vi "Authorize.vi"(6 "timeout (ms) [0: default]":i32, 8 "error in (no error)":errorcluster, 10 "State Parameter":string, 11 "Oauth2 in":refnum<class "Oauth2.lvclass">) -> (0 "error out":errorcluster, 2 "Access Token":string, 3 "Oauth2 out":refnum<class "Oauth2.lvclass">)   [LabVIEW 2013, in "Oauth2.lvclass"]
uses:
  Oauth2.lvclass
  OAuthToken/OAuth2 Token Element -- enum.ctl
  Oauth2.lvclass/Oauth2.ctl
  <vilib>/LabVIEW Open Source Project/OpenURI/uri/URI.lvclass/URI.ctl
  <vilib>/LabVIEW Open Source Project/OpenURI/uri/URI.lvclass
  OAuthToken/OAuthAccessToken.lvclass
  <vilib>/LabVIEW Open Source Project/Connection/Connection.TCP/Connection.TCP.lvclass
  <vilib>/LabVIEW Open Source Project/Connection/Connection/Connection.lvclass
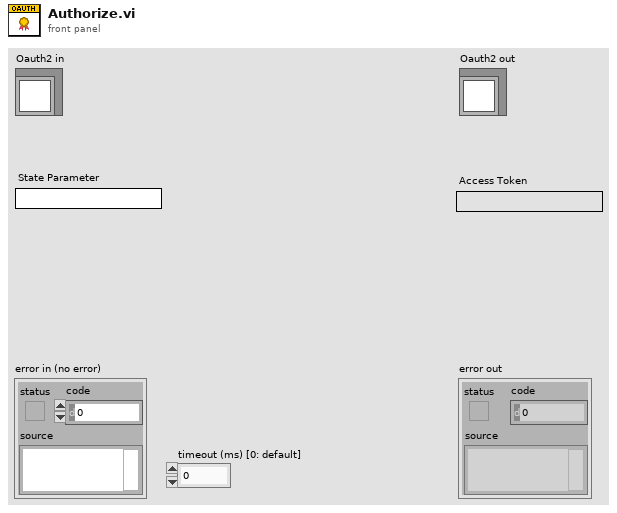
[diagram p1: front panel]
types:
  T1 = typedef "OAuthAccessToken.lvclass/OAuth2 Token Element -- enum.ctl" = enum16{"client_id", "client_secret", "response_type", "scope", "redirect_uri", "error", "error_description", "error_uri", "grant_type", "code", "access_token", "token_type", "expires_in", "username", "password", "refresh_token", "code_challenge", "code_challenge_method", "endpoint element"}
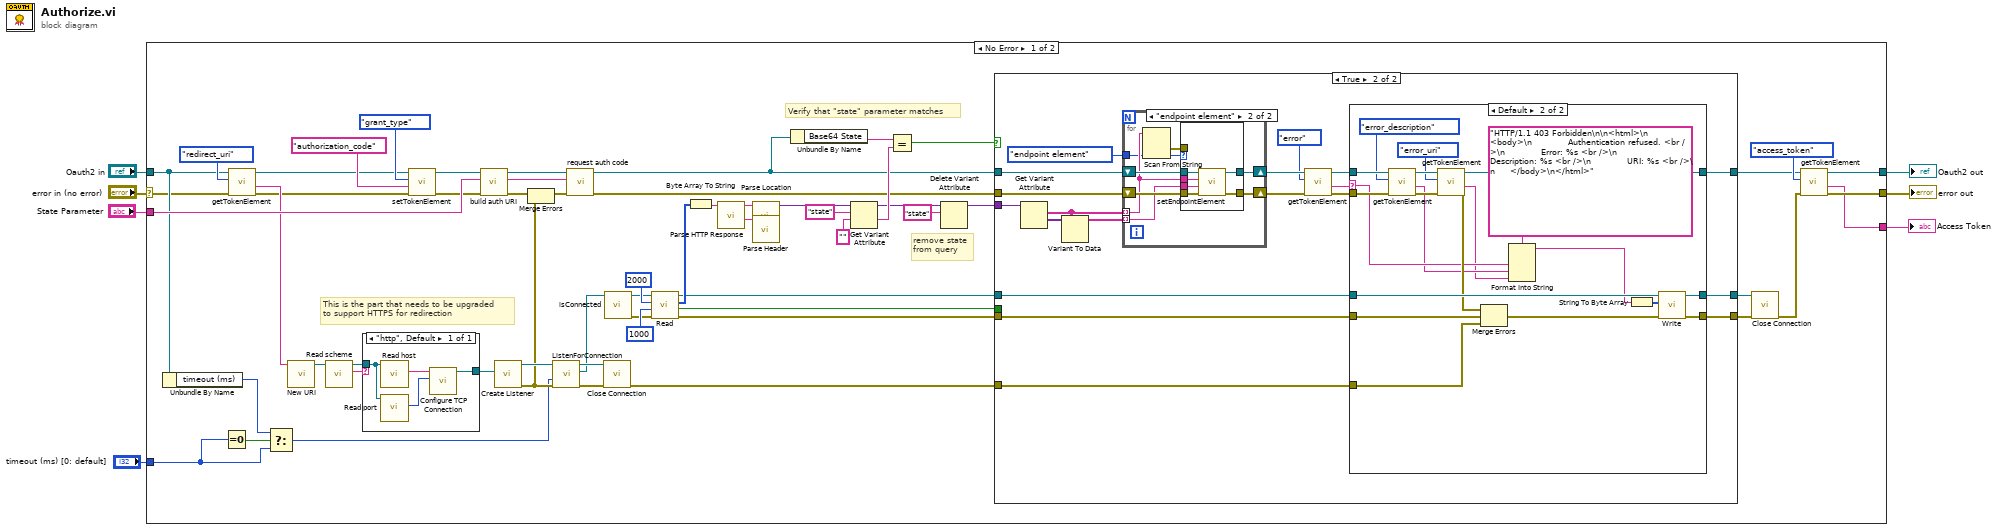
[diagram p0: block diagram]
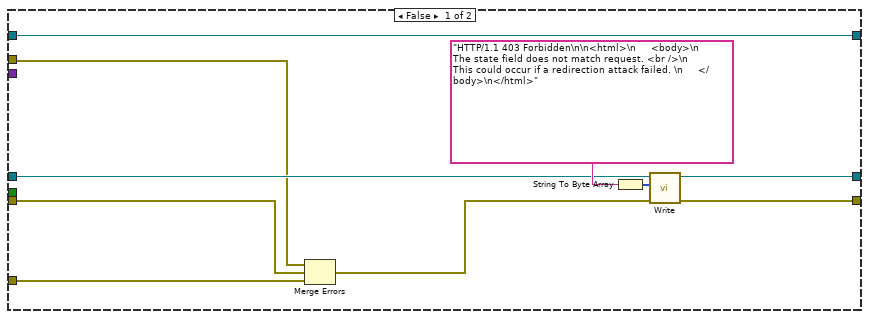
[diagram p2: hidden frame]
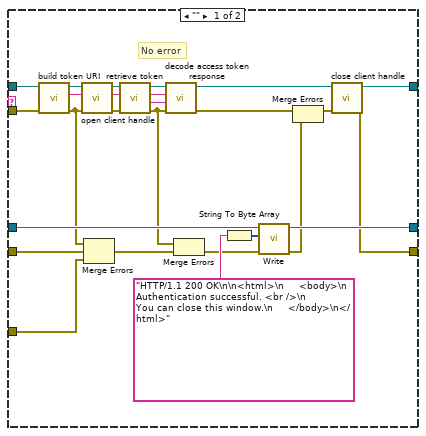
[diagram p3: hidden frame]
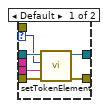
[diagram p4: hidden frame]
diagram:
  n1 = case shown="No Error" "error in (no error)" {
    selector: "error in (no error)" -> [w31 w168]
    tunnel: [w35 w168] -> w6
    tunnel: [w37 w167] -> w4
    tunnel: "Oauth2 in" -> [w32 w167]
    tunnel: "State Parameter" -> [w64 _]
    tunnel: [w27 _] -> w2
    tunnel: "timeout (ms) [0: default]" -> [w10 _]
    frame No Error {
      # "This is the part that needs to be upgraded\nto support HTTPS for redirection"
      # "remove state\nfrom query"
      # "Verify that \"state\" parameter matches"
      n2 = Unbundle By Name(w32) -> ("timeout (ms)"=w43:i32)
      n3 = Equal To 0?(x=w10) -> (x = 0?=w44:bool)
      n4 = call "getTokenElement.vi"("error in (no error)"=w31, "Token element"=OAuth2_Token_Element_--_enum."redirect_uri", "Oauth2 in"=w32) -> ("error out"=w8:errorcluster, "Value"=w30:string, "Oauth2 out"=w9:refnum<class "Oauth2.lvclass">)  [unwired: 5 in, 1 out]
      n5 = Select(t=w43, s=w44, f=w10) -> (s? t:f=w42:i32)
      n6 = call <vilib>:"New URI.vi"("URI"=w30) -> ("URI"=w29:refnum<class "URI.lvclass">)  [unwired: 9 in, 1 out]
      n7 = call <vilib>:"Read scheme.vi"("URI in"=w29) -> ("scheme"=w66:string, "URI out"=w65:refnum<class "URI.lvclass">)  [unwired: 8 in, 1 out]
      n8 = case shown="\"http\", Default" w66 {
        tunnel: w65 -> [w163]
        tunnel: [w164] -> w55
        frame "http", Default {
          n9 = call <vilib>:"Read host.vi"("URI in"=w163) -> ("host"=w166:string)  [unwired: 8 in, 2 out]
          n10 = call <vilib>:"Read port.vi"("URI in"=w163) -> ("port"=w165:u16)  [unwired: 8 in, 2 out]
          n11 = call <vilib>:"Configure TCP Connection.vi"("remote port (80)"=w165, "address (localhost)"=w166) -> ("Connection.TCP"=w164:refnum<class "Connection.TCP.lvclass">)  [unwired: 8 in, 1 out]
        }
      }
      n12 = call "setTokenElement.vi"("error in (no error)"=w8, "Value"="authorization_code", "Token element"=OAuth2_Token_Element_--_enum."grant_type", "Oauth2 in"=w9) -> ("error out"=w11:errorcluster, "Oauth2 out"=w12:refnum<class "Oauth2.lvclass">)  [unwired: 6 in]
      n13 = call "build auth URI.vi"("error in (no error)"=w11, "State Parameter"=w64, "Oauth2 in"=w12) -> ("error out"=w49:errorcluster, "Authorization Request URI"=w51:string, "Oauth2"=w50:refnum<class "Oauth2.lvclass">)  [unwired: 6 in]
      n14 = call <vilib>:"Create Listener.vi"("Connection Configuration"=w55) -> ("error out"=w53:errorcluster, "Listener"=w61:refnum<class "Connection.lvclass">)  [unwired: 9 in]
      n15 = Merge Errors(w49, w53) -> (w52:errorcluster)
      n16 = call <vilib>:"ListenForConnection.vi"("error in (no error)"=w53, "timeout (2000 ms)"=w42, "Listener"=w61) -> ("error out"=w63:errorcluster, "Connection"=w58:refnum<class "Connection.lvclass">, "Listener out"=w60:refnum<class "Connection.lvclass">)  [unwired: 5 in, 1 out]
      n17 = call-dynamic "request auth code.vi"("error in (no error)"=w52, "Request URI"=w51, "Oauth2 in"=w50) -> ("error out"=w18:errorcluster, "Oauth2 out"=w19:refnum<class "Oauth2.lvclass">)  [unwired: 7 in]
      n18 = call <vilib>:"Close Connection.vi"("error in (no error)"=w63, "Connection in"=w60) -> ("error out"=w46:errorcluster)  [unwired: 8 in, 1 out]
      n19 = call <vilib>:"isConnected.vi"("Connection in"=w58) -> ("error out"=w56:errorcluster, "Connection out"=w57:refnum<class "Connection.lvclass">)  [unwired: 8 in, 1 out]
      n20 = call <vilib>:"Read.vi"("error in (no error)"=w56, "timeout (2000 ms)"=1000 ("bytes to read (100)"), "bytes to read (100)"=2000, "TCPConnection in"=w57) -> ("error out"=w45:errorcluster, "timed out"=w38:bool, "Bytes"=w54:u8[], "TCPConnection out"=w47:refnum<class "Connection.lvclass">)  [unwired: 3 in, 1 out]
      n21 = Byte Array To String(unsigned byte array=w54) -> (string=w26:string)
      n22 = call "Parse HTTP Response.vi"("HTTP Response"=w26) -> ("Header"=w25:string, "Location"=w24:string)  [unwired: 5 in, 4 out]
      n23 = call "Parse Location.vi"("Location"=w24) -> ("Query Parameters"=w23:variant)  [unwired: 10 in]
      n24 = call "Parse Header.vi"("HTTP Header"=w25) -> ()  [unwired: 10 in, 1 out]
      n25 = Unbundle By Name(w19) -> ("Base64 State"=w40:string)
      n26 = Get Variant Attribute(Variant=w23, name="state", default value (empty Variant)="") -> (duplicate Variant=w17:variant, value=w20:string)  [unwired: 1 in, 2 out]
      n27 = Equal?(x=w40, y=w20) -> (x = y?=w39:bool)
      n28 = Delete Variant Attribute(6:"state", 7:w17) -> (3:w16:variant)  [unwired: 1 in, 2 out]
      n29 = case shown="True" w39 {
        tunnel: w19 -> [w68 w89]
        tunnel: w18 -> [w67 w88]
        tunnel: [w73 w95] -> w48
        tunnel: w47 -> [w74 w94]
        tunnel: w46 -> [w71 w93]
        tunnel: w45 -> [w70 w92]
        tunnel: [w68 w91] -> w28
        tunnel: [w72 w90] -> w41
        tunnel: w38 -> [_ _]
        tunnel: w16 -> [_ w83]
        frame False {
          n30 = Merge Errors(w67, w70, w71) -> (w69:errorcluster)
          n31 = String To Byte Array(string="HTTP/1.1 403 Forbidden\n\n<html>\n     <body>\n           The state field does not match request. <br />\n           This could occur if a redirection attack failed. \n     </body>\n</html>" ("regular expression")) -> (unsigned byte array=w76:u8[])
          n32 = call <vilib>:"Write.vi"("error in (no error)"=w69, "Bytes"=w76, "Connection in"=w74) -> ("error out"=w72:errorcluster, "Connection"=w73:refnum<class "Connection.lvclass">)  [unwired: 7 in]
        }
        frame True {
          n33 = Get Variant Attribute(Variant=w83) -> (names=w84:string[], values=w86:variant[])  [unwired: 3 in, 2 out]
          n34 = Variant To Data(type=w84, Variant=w86) -> (data=w85:string[])  [unwired: 1 in, 1 out]
          n35 = for {
            shift-right: [w148] -> w82
            shift-left: w89 -> [w149]
            shift-right: [w145] -> w80
            shift-left: w88 -> [w147]
            tunnel: w84 -> [w143] mode=indexing
            tunnel: w85 -> [w146] mode=indexing
            tunnel: OAuth2_Token_Element_--_enum."endpoint element" ("Token element") -> [w142]
            n36 = Scan From String(input string=w143, default 1=w142) -> (error out=w144:errorcluster, output 1=w150:T1)  [unwired: 3 in, 2 out]
            n37 = case shown="\"endpoint element\"" w150 {
              selector: w150 -> [w154 _]
              tunnel: w149 -> [w156 w162]
              tunnel: [w155 w161] -> w148
              tunnel: w147 -> [w153 w160]
              tunnel: w146 -> [w152 w158]
              tunnel: [w151 w159] -> w145
              tunnel: w144 -> [_ _]
              tunnel: w143 -> [_ w157]
              frame Default {
                n38 = call "setTokenElement.vi"("error in (no error)"=w153, "Value"=w152, "Token element"=w154, "Oauth2 in"=w156) -> ("error out"=w151:errorcluster, "Oauth2 out"=w155:refnum<class "Oauth2.lvclass">)  [unwired: 6 in]
              }
              frame "endpoint element" {
                n39 = call "setEndpointElement.vi"("error in (no error)"=w160, "Value"=w158, "Endpoint Name"=w157, "Oauth2 in"=w162) -> ("error out"=w159:errorcluster, "Oauth2 out"=w161:refnum<class "Oauth2.lvclass">)  [unwired: 6 in]
              }
            }
          }
          n40 = call "getTokenElement.vi"("error in (no error)"=w80, "Token element"=OAuth2_Token_Element_--_enum."error", "Oauth2 in"=w82) -> ("error out"=w79:errorcluster, "Value"=w77:string, "Oauth2 out"=w81:refnum<class "Oauth2.lvclass">)  [unwired: 5 in, 1 out]
          n41 = case shown="Default" w77 {
            selector: w77 -> [_ w126]
            tunnel: [w121 w141] -> w95
            tunnel: w94 -> [w118 w139]
            tunnel: w93 -> [w117 w138]
            tunnel: w92 -> [w116 w137]
            tunnel: [w109 w131] -> w91
            tunnel: [w98 w136] -> w90
            tunnel: w81 -> [w97 w134]
            tunnel: w79 -> [w96 w129]
            frame "" {
              # "No error"
              n42 = call-dynamic "build token URI.vi"("error in (no error)"=w96, "Oauth2 in"=w97) -> ("error out"=w111:errorcluster, "Token Request URI"=w112:string, "Oauth2"=w113:refnum<class "Oauth2.lvclass">)  [unwired: 7 in]
              n43 = call "open client handle.vi"("error in (no error)"=w111, "Request URI in"=w112, "Oauth2 in"=w113) -> ("error out"=w107:errorcluster, "Request URI dup"=w106:string, "Oauth2 out"=w108:refnum<class "Oauth2.lvclass">)  [unwired: 6 in]
              n44 = Merge Errors(w111, w116, w117) -> (w115:errorcluster)
              n45 = call "retrieve token.vi"("error in (no error)"=w107, "Token Request URI"=w106, "Oauth2 in"=w108) -> ("error out"=w103:errorcluster, "Response"=w100:string, "Header"=w101:string, "Oauth2 out"=w105:refnum<class "Oauth2.lvclass">)  [unwired: 5 in]
              n46 = call-dynamic "decode access token response.vi"("error in (no error)"=w103, "Response"=w100, "Header"=w101, "Oauth2 in"=w105) -> ("error out"=w102:errorcluster, "Oauth2"=w104:refnum<class "Oauth2.lvclass">)  [unwired: 6 in]
              n47 = Merge Errors(w103, w115) -> (w114:errorcluster)
              n48 = String To Byte Array(string="HTTP/1.1 200 OK\n\n<html>\n     <body>\n            Authentication successful. <br />\n            You can close this window.\n     </body>\n</html>" ("regular expression")) -> (unsigned byte array=w120:u8[])
              n49 = call <vilib>:"Write.vi"("error in (no error)"=w114, "Bytes"=w120, "Connection in"=w118) -> ("error out"=w99:errorcluster, "Connection"=w121:refnum<class "Connection.lvclass">)  [unwired: 7 in]
              n50 = Merge Errors(w102, w99) -> (w110:errorcluster)
              n51 = call "close client handle.vi"("error in (no error)"=w110, "Oauth2 in"=w104) -> ("error out"=w98:errorcluster, "Oauth2 out"=w109:refnum<class "Oauth2.lvclass">)  [unwired: 8 in]
            }
            frame Default {
              n52 = call "getTokenElement.vi"("error in (no error)"=w129, "Token element"=OAuth2_Token_Element_--_enum."error_description", "Oauth2 in"=w134) -> ("error out"=w130:errorcluster, "Value"=w125:string, "Oauth2 out"=w132:refnum<class "Oauth2.lvclass">)  [unwired: 5 in, 1 out]
              n53 = call "getTokenElement.vi"("error in (no error)"=w130, "Token element"=OAuth2_Token_Element_--_enum."error_uri", "Oauth2 in"=w132) -> ("error out"=w128:errorcluster, "Value"=w124:string, "Oauth2 out"=w131:refnum<class "Oauth2.lvclass">)  [unwired: 5 in, 1 out]
              n54 = Merge Errors(w128, w137, w138) -> (w135:errorcluster)
              n55 = Format Into String(format string="HTTP/1.1 403 Forbidden\n\n<html>\n     <body>\n            Authentication refused. <br />\n            Error: %s <br />\n            Description: %s <br />\n            URI: %s <br />\n     </body>\n</html>" ("regular expression"), w126, w125, w124) -> (resulting string=w123:string)  [unwired: 2 in, 1 out]
              n56 = String To Byte Array(string=w123) -> (unsigned byte array=w140:u8[])
              n57 = call <vilib>:"Write.vi"("error in (no error)"=w135, "Bytes"=w140, "Connection in"=w139) -> ("error out"=w136:errorcluster, "Connection"=w141:refnum<class "Connection.lvclass">)  [unwired: 7 in]
            }
          }
        }
      }
      n58 = call <vilib>:"Close Connection.vi"("error in (no error)"=w41, "Connection in"=w48) -> ("error out"=w36:errorcluster)  [unwired: 8 in, 1 out]
      n59 = call "getTokenElement.vi"("error in (no error)"=w36, "Token element"=OAuth2_Token_Element_--_enum."access_token", "Oauth2 in"=w28) -> ("error out"=w35:errorcluster, "Value"=w27:string, "Oauth2 out"=w37:refnum<class "Oauth2.lvclass">)  [unwired: 5 in, 1 out]
    }
    frame Error {
    }
  }
  "error out" <- w6
  "Oauth2 out" <- w4
  "Access Token" <- w2
